vi "Status Output Loop.vi"(8 "error in (no error)":errorcluster, 11 "CLI in":refnum<class "CLI.lvclass">) -> (0 "error out":errorcluster, 3 "CLI out":refnum<class "CLI.lvclass">)   [LabVIEW 2020, in "neg-pkg-cli.lvlib" / "CLI.lvclass"]
uses:
  CLI.lvclass
  CLI.lvclass/CLI.ctl
  build/ppl/neg-pkg.lvlibp/Status/Status.lvclass
  MGI Console/Source/Console/Console.lvclass
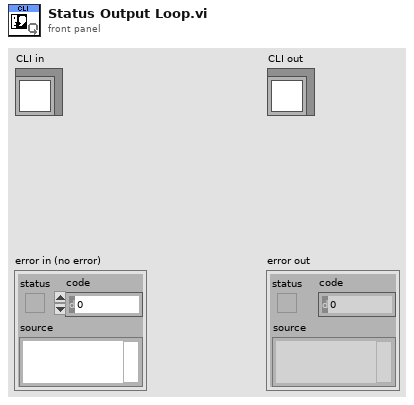
[diagram p1: front panel]
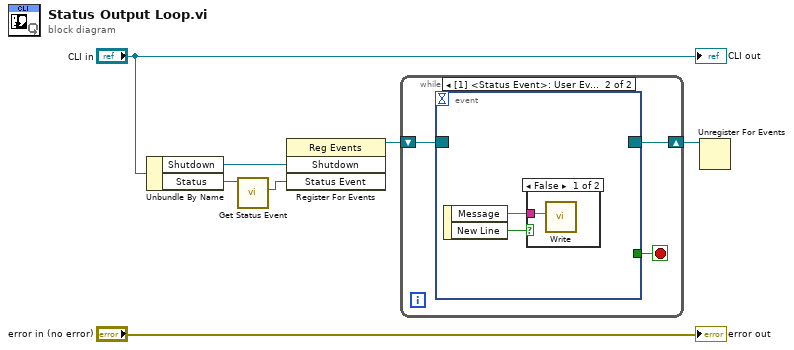
[diagram p0: block diagram]
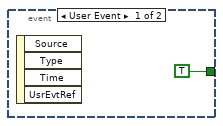
[diagram p2: hidden frame]
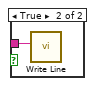
[diagram p3: hidden frame]
diagram:
  n1 = Unbundle By Name("CLI in") -> ("Shutdown"=w3:refnum<user-event>, "Status"=w5:refnum<class "Status.lvclass">)
  n2 = call "Get Status Event.vi"("Status in"=w5) -> ("Status Event"=w4:refnum<user-event>)  [unwired: 8 in, 2 out]
  n3 = register-events(w3, w4) -> (reference out=w2:refnum<event-registration>)  [unwired: 2 in, 1 out]
  n4 = while {
    shift-right: [w8] -> w1
    shift-left: w2 -> [w10]
    stop <- w9 stop-if-true
    n5 = event shown="[1] <Status Event>: User Event" {
      selector: w10 -> [_ _]
      dyn-events: [_ _] -> w8
      timeout: _ -> [_ _]
      tunnel: [TRUE _] -> w9
      event User Event {
        n6 = event-data() -> ()  [unwired: 1 in, 4 out]
      }
      event User Event {
        n7 = event-data() -> ("Message"=w13:string, "New Line"=w12:bool)  [unwired: 1 in]
        n8 = case shown="False" w12 {
          tunnel: w13 -> [w14 w15]
          frame False {
            n9 = call "Write.vi"("String"=w14) -> ()  [unwired: 10 in, 1 out]
          }
          frame True {
            n10 = call "Write Line.vi"("Line"=w15) -> ()  [unwired: 10 in, 1 out]
          }
        }
      }
    }
  }
  n11 = Unregister For Events(event registration refnum=w1) -> ()  [unwired: 1 in, 1 out]
  "error out" <- "error in (no error)"
  "CLI out" <- "CLI in"
